vi "spectrum.vi"(10 "im":dbl[](array[numeric]), 11 "re":dbl[](array[numeric])) -> (3 "spectrum":dbl[](array[numeric]))   [LabVIEW 2020]
uses:
  <vilib>/Analysis/2dsp.llb/Complex FFT.vi
  <vilib>/Analysis/NI_AALPro.lvlib
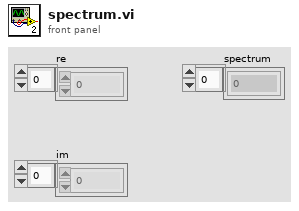
[diagram p1: front panel]
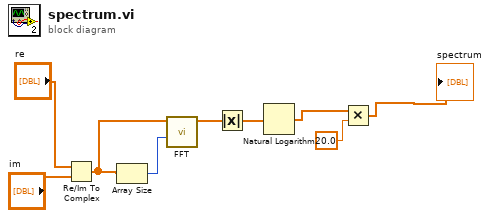
[diagram p0: block diagram]
diagram:
  n1 = Re/Im To Complex(1:"im", 2:"re") -> (0:w3:cdb[])
  n2 = Array Size(array=w3) -> (size(s)=w1:i32)
  n3 = call-poly <vilib>:"FFT.vi"("FFT size"=w1, "X"=w3) -> ("FFT {X}"=w2:cdb[])  [unwired: 8 in, 1 out]
  n4 = Absolute Value(x=w2) -> (abs(x)=w4:dbl[])
  n5 = Natural Logarithm(1:w4) -> (0:w7:dbl[])
  n6 = Multiply(x=w7, y=20.0 ("x")) -> (x*y=→"spectrum":dbl[])
